vi "Write Allow to Close.vi"(8 "error in (no error)":errorcluster, 10 "Allow to close?":bool, 11 "Dialog.lvclass in":refnum<class "Dialog.lvclass">) -> (0 "error out":errorcluster, 3 "Dialog.lvclass out":refnum<class "Dialog.lvclass">)   [LabVIEW 2012, in "Dialog.lvlib" / "Dialog.lvclass"]
uses:
  Dialog.lvclass
  Dialog.lvclass/Dialog.ctl
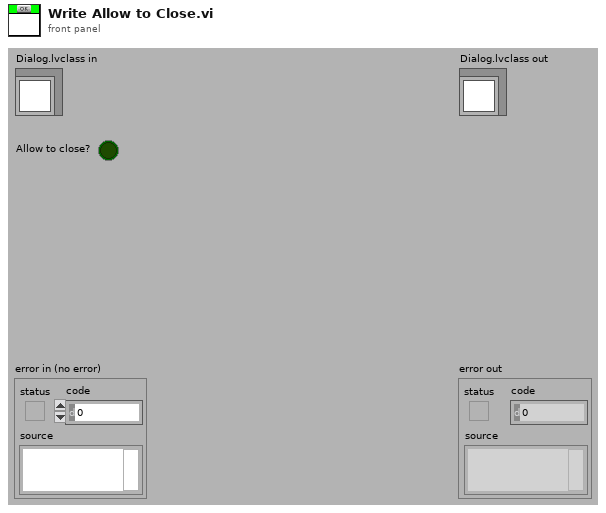
[diagram p1: front panel]
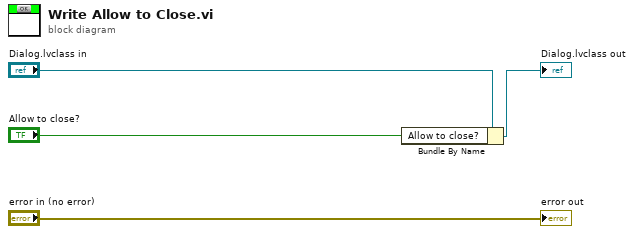
[diagram p0: block diagram]
diagram:
  n1 = Bundle By Name(cluster="Dialog.lvclass in", "Allow to close?"="Allow to close?") -> (→"Dialog.lvclass out":refnum<class "Dialog.lvclass">)
  "error out" <- "error in (no error)"
